vi "Device.Init.vi"(8 "error in (no error)":errorcluster, 11 "SMU.Keithley2600":refnum<class "SMU.Keithley2600.lvclass">) -> (0 "error out":errorcluster, 2 "Result":bool, 3 "SMU.Keithley2600 out":refnum<class "SMU.Keithley2600.lvclass">)   [LabVIEW 2017, in "SMU.Keithley2600.lvclass"]
doc: "---------------------------------------------------------------\nJKI State Machine Objects™\nhttp://jki.net/state-machine-objects/\nCopyright (C) 2005-2015, JKI <info@jki.net>\nALL RIGHTS RESERVEDJKI State Machine Objects (SMO) 1.0.0.5\nJKI - JKI\nCopyright (c) 2016, JKI"
uses:
  SMU.Keithley2600.lvclass
  Typedefs/Resource--Cluster.ctl
  <instrlib>/Keithley 2600 Series/Keithley 2600 Series.lvlib
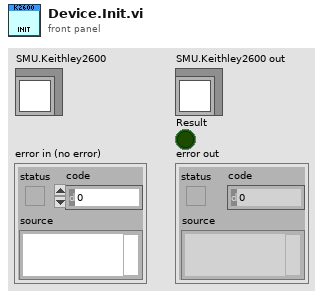
[diagram p1: front panel]
types:
  T1 = typedef "SMU.Keithley2600.lvclass/Resource--Cluster.ctl" = cluster{"VISA resource":refnum<visa-resource-name>, "Channel":i32}
  T2 = typedef "SMU.lvclass/Configuration--Cluster.ctl" = cluster{"VISA Resource":string, "Channel":string}
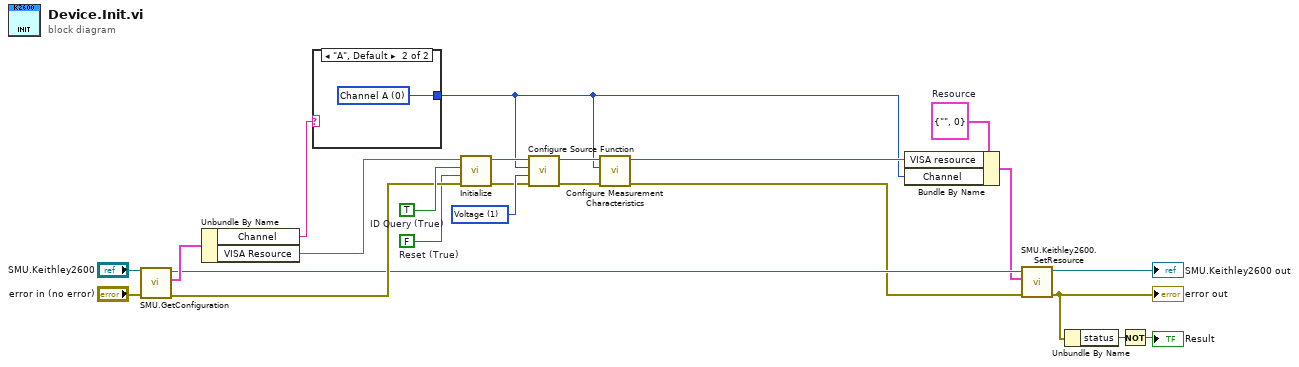
[diagram p0: block diagram]
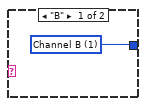
[diagram p2: hidden frame]
diagram:
  w4 = T1 {"VISA resource"="", "Channel"=0}  # Resource
  w8 = 1 items=["Current", "Voltage"] ("Source Function (1: Voltage)")
  w10 = FALSE  # Reset (True)
  w19 = TRUE  # ID Query (True)
  n1 = call-dynamic "SMU.GetConfiguration.vi"("error in (no error)"="error in (no error)", "SMU"="SMU.Keithley2600") -> ("error out"=w18:errorcluster, "Configuration"=w20:T2, "SMU out"=w17:refnum<class "SMU.Keithley2600.lvclass">)  [unwired: 7 in]
  n2 = Unbundle By Name(w20) -> ("Channel"=w14:string, "VISA Resource"=w15:string)
  n3 = case shown="\"A\", Default" w14 {
    tunnel: [w24 w25] -> w2
    frame "B" {
      w24 = 1 items=["Channel A", "Channel B"] ("Source Measure Unit Channel (0: Channel A)")
    }
    frame "A", Default {
      w25 = 0 items=["Channel A", "Channel B"] ("Source Measure Unit Channel (0: Channel A)")
    }
  }
  n4 = call <instrlib>:"Initialize.vi"("error in (no error)"=w18, "Reset (True)"=w10, "ID Query (True)"=w19, "VISA resource name"=w15) -> ("error out"=w7:errorcluster, "VISA resource name out"=w9:refnum<visa-resource-name>)  [unwired: 2 in, 4 out]
  n5 = call <instrlib>:"Configure Source Function.vi"("error in (no error)"=w7, "Source Function (1: Voltage)"=w8, "Source Measure Unit Channel (0: Channel A)"=w2, "VISA resource name"=w9) -> ("error out"=w5:errorcluster, "VISA resource name out"=w6:refnum<visa-resource-name>)  [unwired: 6 in]
  n6 = call <instrlib>:"Configure Measurement Characteristics.vi"("error in (no error)"=w5, "Source Measure Unit Channel (0: Channel A)"=w2, "VISA resource name"=w6) -> ("error out"=w1:errorcluster, "VISA resource name out"=w3:refnum<visa-resource-name>)  [unwired: 7 in]
  n7 = Bundle By Name(cluster=w4, "VISA resource"=w3, "Channel"=w2) -> (w16:T1)
  n8 = call "SMU.Keithley2600.SetResource.vi"("error in (no error)"=w1, "Resource"=w16, "SMU.Keithley2600 in"=w17) -> ("error out"=w11:errorcluster, "SMU.Keithley2600 out"=→"SMU.Keithley2600 out":refnum<class "SMU.Keithley2600.lvclass">)  [unwired: 7 in]
  "error out" <- w11
  n9 = Unbundle By Name(w11) -> ("status"=w13:bool)
  n10 = Not(x=w13) -> (.not. x?=→"Result":bool)
